vi "Scatter2000.vi"   [LabVIEW 2013]
uses:
  <vilib>/Heliosphere Research LLC/Advanced Plotting Toolkit/Advanced Plotting Toolkit.lvlib
types:
  T1 = typedef "Advanced Plotting Toolkit.lvlib/PlotID.ctl" = i32
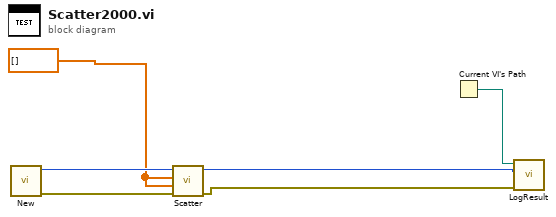
[diagram p0: block diagram]
diagram:
  w1 = dbl[] [] ("X Data")
  n1 = call <vilib>:"New.vi"() -> ("error out"=w4:errorcluster, "Plot ID"=w5:T1)  [unwired: 10 in]
  n2 = call <vilib>:"Scatter.vi"("error in (no error)"=w4, "Y Data"=w1, "X Data"=w1, "Plot ID"=w5) -> ("error out"=w2:errorcluster, "Plot ID Out"=w3:T1)  [unwired: 6 in]
  n3 = Current VI's Path() -> (path=w6:path)
  n4 = call "LogResult.vi"("Test Result"=w2, "Test Artifact"=w3, "VI Path"=w6) -> ()  [unwired: 9 in]
